vi "F Dwf Analog IO Channel Name.vi"(7 "szLabel":string, 8 "error in (no error)":errorcluster, 9 "szName":string, 10 "idxChannel":i32, 11 "hdwf":i32) -> (0 "error out":errorcluster, 1 "szName out":string, 3 "function return":i32, 5 "szLabel out":string)   [LabVIEW 2019, in "Olasdwf.lvlib"]
doc: "DWFAPI int FDwfAnalogIOChannelName(HDWF hdwf, int idxChannel, char szName[32], char szLabel[16]);"
uses:
  Olasdwf.lvlib
  Windows/System32/dwf.dll
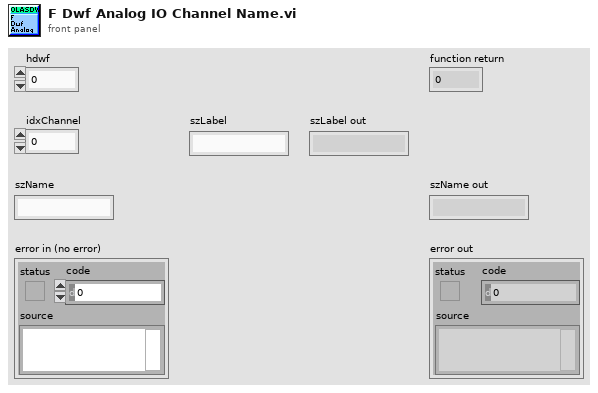
[diagram p1: front panel]
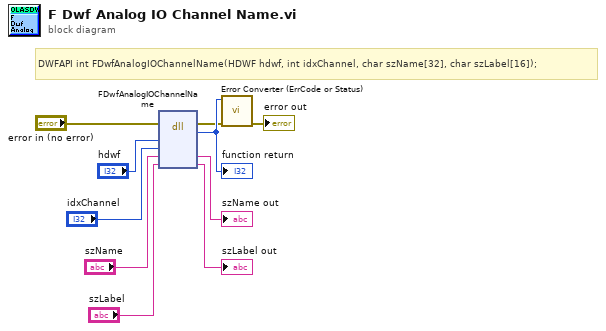
[diagram p0: block diagram]
diagram:
  # "DWFAPI int FDwfAnalogIOChannelName(HDWF hdwf, int idxChannel, char szName[32], char szLabel[16]);"
  n1 = dll-call lib="C:/Windows/System32/dwf.*" fn="FDwfAnalogIOChannelName"(error in="error in (no error)", "hdwf"="hdwf", "idxChannel"="idxChannel", "szName"="szName", "szLabel"="szLabel") -> (error out=w2:errorcluster, w10:i32, "szName"=→"szName out":string, "szLabel"=→"szLabel out":string)  [unwired: 4 in, 1 out]
  "function return" <- w10
  n2 = call "Error Converter (ErrCode or Status).vi"("error in (no error)"=w2, "error code"=w10) -> ("error out"=→"error out":errorcluster)  [unwired: 9 in]
